vi "WindSIM.vi"() -> ()   [LabVIEW 2019]
uses:
  <vilib>/Utility/miscctls.llb/LV3DPointTypeDef.ctl
  <vilib>/picture/3D Picture Control/Object/Create Object (drawable).vi
  <vilib>/picture/3D Picture Control/Object/Add Object (no reference).vi
  <vilib>/picture/3D Picture Control/NI_3D Picture Control.lvlib
panel:
  in  "Activate Rotation?":bool
  in  "Turbine Speed %":dbl(slide) scale=0.0..100.0
  out "3D Picture":refnum<vi>(3d-picture)
  in  "Pitch Value":dbl(slide) scale=-20.0..20.0
  in  "Tab Control":T1(tab)
  in  "Blade1 Translation":cluster{"X":sgl, "Y":sgl, "Z":sgl}={"X"=2.0, "Y"=1.5, "Z"=0.0}
  in  "Blade1 Angle":dbl=127.0
  in  "Blade2 Translation":cluster{"X":sgl, "Y":sgl, "Z":sgl}={"X"=-2.0, "Y"=1.5, "Z"=0.0}
  in  "Blade2 Angle":sgl=235.0
  in  "Blade3 Transalation":cluster{"X":sgl, "Y":sgl, "Z":sgl}={"X"=0.0, "Y"=-2.5, "Z"=0.0}
  in  "Blade3 Angle":sgl
  in  "Nacele R":sgl=1.0 min=0.1 max=100
  in  "Length X":sgl=0.5
  in  "Length Y":sgl=3.0
  in  "Length Z":sgl=0.2
  in  "Length":sgl=2.0
  in  "Radius":sgl=0.001
  in  "Coeff":sgl=0.39999998
  in  "Character Size":sgl=0.2
  in  "Rotation Axis":cluster{"X":sgl, "Y":sgl, "Z":sgl}={"X"=0.0, "Y"=1.0, "Z"=0.0}
  in  "Camera Position":T2={"X"=0.0, "Y"=0.0, "Z"=6.0}
  in  "Up Direction":T2={"X"=0.0, "Y"=1.0, "Z"=0.0}
  in  "Target":T2
  out "error out":errorcluster
  in  "stop":bool
  # "Controls: Hold Shift + Mouse IN/OUT to ZOOM\n              Hold CTRL + Mouse IN/OUT to Move"
  # "Blade parameters"
  # "Axis parameters"
  # "Zoom coeff"
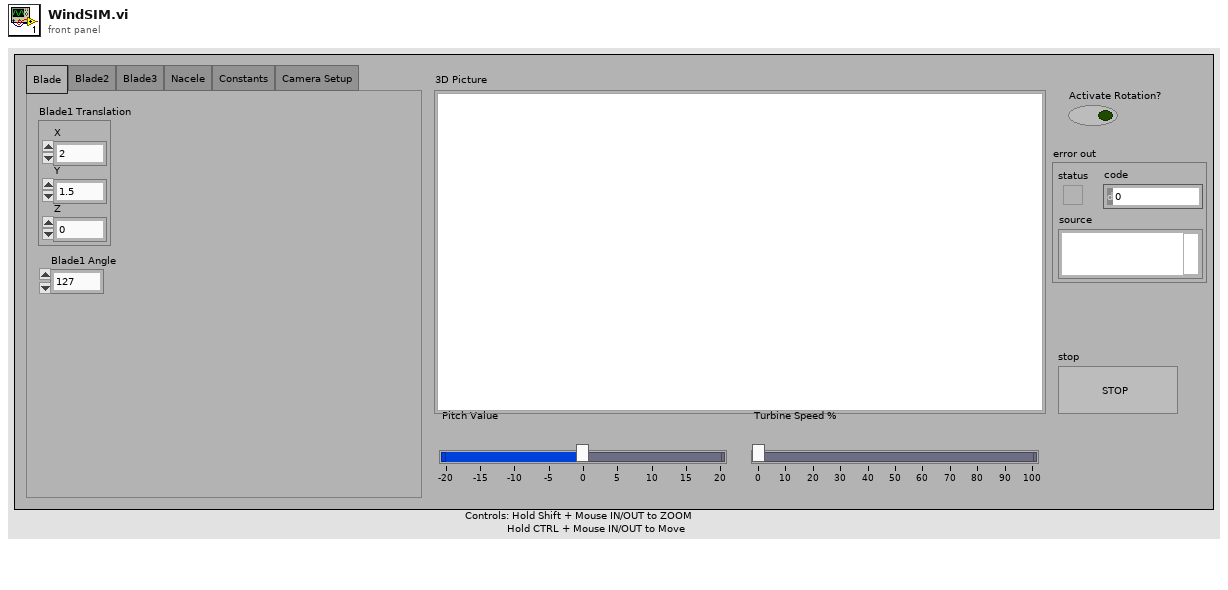
[diagram p1: front panel]
types:
  T1 = enum32{"Blade", "Blade2", "Blade3", "Nacele", "Constants", "Camera Setup"}
  T2 = typedef "LV3DPointTypeDef.ctl" = cluster{"X":sgl, "Y":sgl, "Z":sgl}
  T3 = cluster{"Red":sgl, "Green":sgl, "Blue":sgl, "Alpha":sgl}
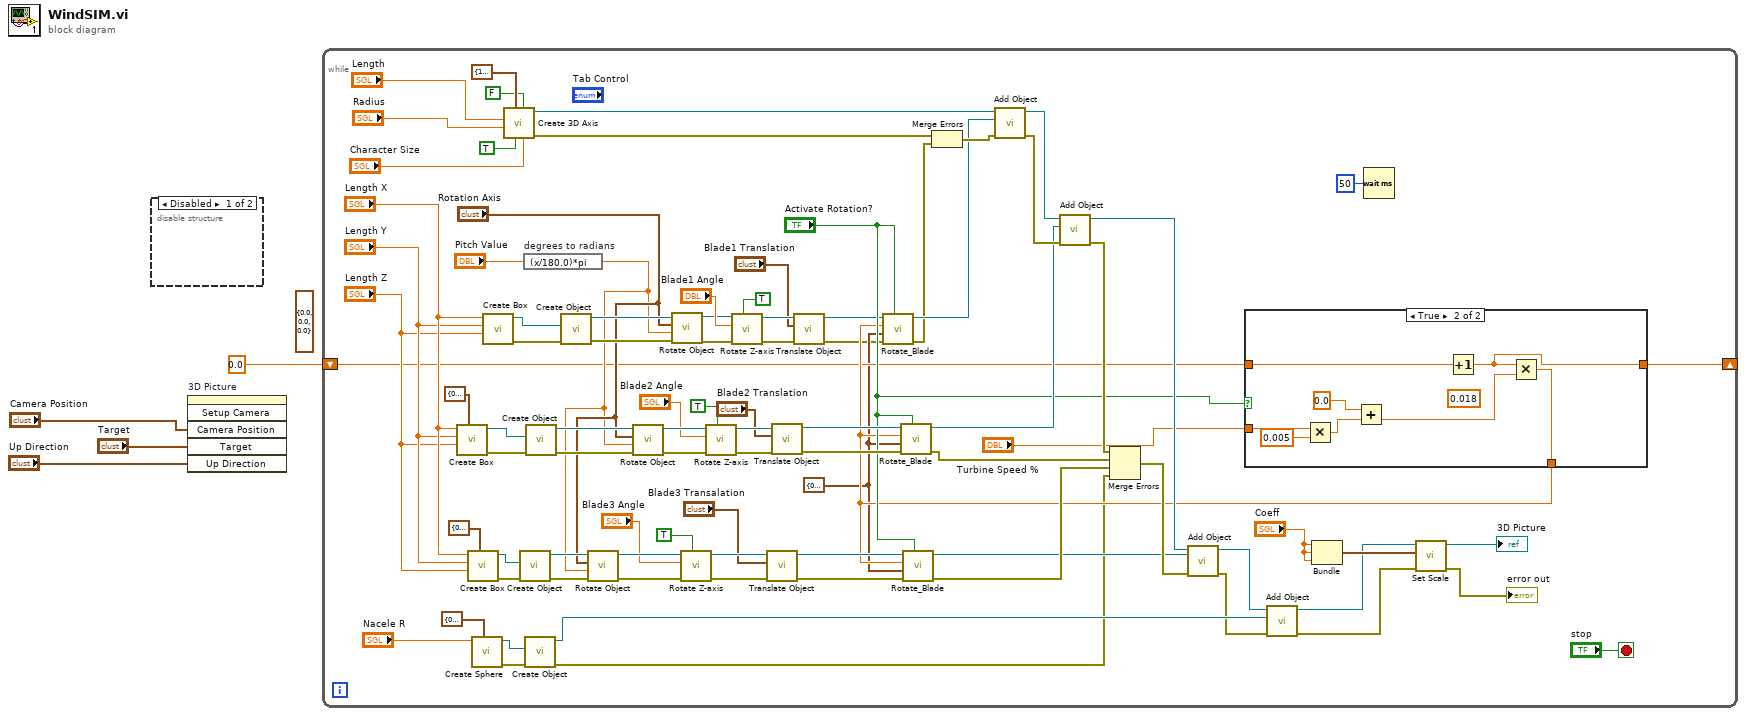
[diagram p0: block diagram]
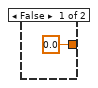
[diagram p3: hidden frame]
diagram:
  (unwired) cluster{dbl, dbl, "Turbine Speed %":dbl} {0.0, 0.0, "Turbine Speed %"=0.0}
  n1 = disable-structure shown="Disabled" {
    frame Disabled {
    }
    frame Enabled {
    }
  }
  n2 = invoke on="3D Picture" class="SceneGraphDisp (strict)" method="Setup Camera"("Camera Position"="Camera Position", "Target"="Target", "Up Direction"="Up Direction") -> ()  [unwired: 3 in, 6 out]
  n3 = while {
    shift-right: [w9] -> _
    shift-left: 0.0 -> [w22]
    stop <- "stop" stop-if-true
    w21 = cluster{"X":sgl, "Y":sgl, "Z":sgl} {"X"=0.0, "Y"=0.0, "Z"=1.0} ("Axis")
    n4 = call <vilib>:"Create Box.vi"("Color"=T3 {"Red"=0.0, "Green"=1.0, "Blue"=0.0, "Alpha"=1.0}, "Length Z"="Length Z", "Length Y"="Length Y", "Length X"="Length X") -> ("error out"=w66:errorcluster, "New Box Refnum"=w68:refnum<vi>)  [unwired: 6 in]
    n5 = call <vilib>:"Create Box.vi"("Color"=T3 {"Red"=0.0, "Green"=0.0, "Blue"=1.0, "Alpha"=1.0}, "Length Z"="Length Z", "Length Y"="Length Y", "Length X"="Length X") -> ("error out"=w54:errorcluster, "New Box Refnum"=w55:refnum<vi>)  [unwired: 6 in]
    n6 = call <vilib>:"Create Sphere.vi"("Color"=T3 {"Red"=0.0, "Green"=1.0, "Blue"=1.0, "Alpha"=1.0}, "Radius"="Nacele R") -> ("error out"=w17:errorcluster, "New Sphere Refnum"=w18:refnum<vi>)  [unwired: 8 in]
    n7 = call <vilib>:"Create Box.vi"("Length Z"="Length Z", "Length Y"="Length Y", "Length X"="Length X") -> ("error out"=w77:errorcluster, "New Box Refnum"=w76:refnum<vi>)  [unwired: 7 in]
    n8 = call <vilib>:"Create 3D Axis.vi"("Character Size"="Character Size", "Half plane?"=FALSE, "Axis label?"=TRUE, "Color"=T3 {"Red"=1.0, "Green"=0.0, "Blue"=0.0, "Alpha"=1.0}, "Radius"="Radius", "Length"="Length") -> ("error out"=w84:errorcluster, "New Object Refnum"=w92:refnum<vi>)  [unwired: 4 in]
    n9 = call-poly <vilib>:"Create Object.vi"("error in (no error)"=w54, "Geometry"=w55) -> ("error out"=w52:errorcluster, "Scene:New Object"=w53:refnum<vi>)  [unwired: 8 in]
    n10 = expression code="(x/180.0)*pi" "degrees to radians"("Pitch Value") -> (w41:dbl)
    n11 = call-poly <vilib>:"Create Object.vi"("error in (no error)"=w17, "Geometry"=w18) -> ("error out"=w11:errorcluster, "Scene:New Object"=w14:refnum<vi>)  [unwired: 8 in]
    n12 = call-poly <vilib>:"Create Object.vi"("error in (no error)"=w66, "Geometry"=w68) -> ("error out"=w65:errorcluster, "Scene:New Object"=w67:refnum<vi>)  [unwired: 8 in]
    n13 = call-poly <vilib>:"Create Object.vi"("error in (no error)"=w77, "Geometry"=w76) -> ("error out"=w74:errorcluster, "Scene:New Object"=w75:refnum<vi>)  [unwired: 8 in]
    n14 = call <vilib>:"Rotate Object.vi"("error in (no error)"=w52, "Angle"=w41, "Axis"="Rotation Axis", "Scene.Object In"=w53) -> ("error out"=w50:errorcluster, "Scene.Object Out"=w51:refnum<vi>)  [unwired: 6 in]
    n15 = call <vilib>:"Rotate Object.vi"("error in (no error)"=w65, "Angle"=w41, "Axis"="Rotation Axis", "Scene.Object In"=w67) -> ("error out"=w64:errorcluster, "Scene.Object Out"=w63:refnum<vi>)  [unwired: 6 in]
    n16 = call <vilib>:"Rotate Object.vi"("error in (no error)"=w74, "Angle"=w41, "Axis"="Rotation Axis", "Scene.Object In"=w75) -> ("error out"=w71:errorcluster, "Scene.Object Out"=w72:refnum<vi>)  [unwired: 6 in]
    n17 = call <vilib>:"Rotate Z-axis.vi"("Relative?"=TRUE, "error in (no error)"=w50, "angle"="Blade3 Angle", "Scene Object In"=w51) -> ("error out"=w48:errorcluster, "Scene Object Out"=w49:refnum<vi>)  [unwired: 6 in]
    n18 = call <vilib>:"Rotate Z-axis.vi"("Relative?"=TRUE, "error in (no error)"=w64, "angle"="Blade2 Angle", "Scene Object In"=w63) -> ("error out"=w61:errorcluster, "Scene Object Out"=w62:refnum<vi>)  [unwired: 6 in]
    n19 = call <vilib>:"Rotate Z-axis.vi"("Relative?"=TRUE, "error in (no error)"=w71, "angle"="Blade1 Angle", "Scene Object In"=w72) -> ("error out"=w69:errorcluster, "Scene Object Out"=w70:refnum<vi>)  [unwired: 6 in]
    n20 = call <vilib>:"Translate Object.vi"("error in (no error)"=w48, "Translation"="Blade3 Transalation", "Scene.Object In"=w49) -> ("error out"=w31:errorcluster, "Scene.Object Out"=w32:refnum<vi>)  [unwired: 7 in]
    n21 = call <vilib>:"Translate Object.vi"("error in (no error)"=w61, "Translation"="Blade2 Translation", "Scene.Object In"=w62) -> ("error out"=w33:errorcluster, "Scene.Object Out"=w34:refnum<vi>)  [unwired: 7 in]
    n22 = call <vilib>:"Translate Object.vi"("error in (no error)"=w69, "Translation"="Blade1 Translation", "Scene.Object In"=w70) -> ("error out"=w6:errorcluster, "Scene.Object Out"=w7:refnum<vi>)  [unwired: 7 in]
    n23 = case shown="True" "Activate Rotation?" {
      tunnel: w22 -> [_ w102]
      tunnel: [0.0 w101] -> w9
      tunnel: [_ w100] -> w23
      tunnel: "Turbine Speed %" -> [_ w99]
      frame False {
      }
      frame True {
        (unwired) 0.018 ("y")
        n24 = Multiply(x=w99, y=0.005) -> (x*y=w97:dbl)
        n25 = Add(x=0.0, y=w97) -> (x+y=w96:dbl)
        n26 = Increment(x=w102) -> (x+1=w101:dbl)
        n27 = Multiply(x=w101, y=w96) -> (x*y=w100:dbl)
      }
    }
    n28 = call "Rotate_Blade.vi"("Activate Rotation?"="Activate Rotation?", "error in"=w6, "Axis"=w21, "angle"=w23, "Scene Object In"=w7) -> ("error out"=w29:errorcluster, "Scene Object Out"=w30:refnum<vi>)  [unwired: 5 in]
    n29 = call "Rotate_Blade.vi"("Activate Rotation?"="Activate Rotation?", "error in"=w33, "Axis"=w21, "angle"=w23, "Scene Object In"=w34) -> ("error out"=w28:errorcluster, "Scene Object Out"=w25:refnum<vi>)  [unwired: 5 in]
    n30 = call "Rotate_Blade.vi"("Activate Rotation?"="Activate Rotation?", "error in"=w31, "Axis"=w21, "angle"=w23, "Scene Object In"=w32) -> ("error out"=w27:errorcluster, "Scene Object Out"=w26:refnum<vi>)  [unwired: 5 in]
    n31 = Merge Errors(w84, w29) -> (w83:errorcluster)
    n32 = call-poly <vilib>:"Add Object.vi"("error in (no error)"=w83, "New Object In"=w30, "Scene Object In"=w92) -> ("error out"=w38:errorcluster, "Scene Object Out"=w56:refnum<vi>)  [unwired: 7 in]
    n33 = call-poly <vilib>:"Add Object.vi"("error in (no error)"=w38, "New Object In"=w25, "Scene Object In"=w56) -> ("error out"=w35:errorcluster, "Scene Object Out"=w36:refnum<vi>)  [unwired: 7 in]
    n34 = Merge Errors(w35, w28, w27, w11) -> (w37:errorcluster)
    n35 = call-poly <vilib>:"Add Object.vi"("error in (no error)"=w37, "New Object In"=w26, "Scene Object In"=w36) -> ("error out"=w10:errorcluster, "Scene Object Out"=w15:refnum<vi>)  [unwired: 7 in]
    n36 = call-poly <vilib>:"Add Object.vi"("error in (no error)"=w10, "New Object In"=w14, "Scene Object In"=w15) -> ("error out"=w13:errorcluster, "Scene Object Out"=w12:refnum<vi>)  [unwired: 7 in]
    n37 = Bundle("Coeff"="Coeff", "Coeff"="Coeff", "Coeff"="Coeff") -> (w16:cluster{"Coeff":sgl, "Coeff":sgl, "Coeff":sgl})  [unwired: 1 in]
    n38 = Wait (ms)(milliseconds to wait=u32 50) -> ()  [unwired: 1 out]
    n39 = call <vilib>:"Set Scale.vi"("error in (no error)"=w13, "Scale"=w16, "Scene Object"=w12) -> ("error out"=→"error out":errorcluster, "Scaled Object"=→"3D Picture":refnum<vi>)  [unwired: 7 in]
  }
